vi "1.dé_electronique_Led_Boucle_GJE.vi"() -> ()   [LabVIEW 2018]
panel:
  in  "Numérique":i8=1 min=1 max=6
  out "7":bool
  out "3":bool
  out "2":bool
  out "6":bool
  out "4":bool
  out "1":bool
  out "5":bool
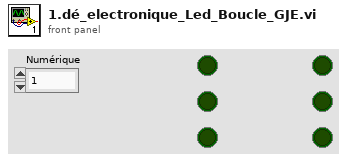
[diagram p1: front panel]
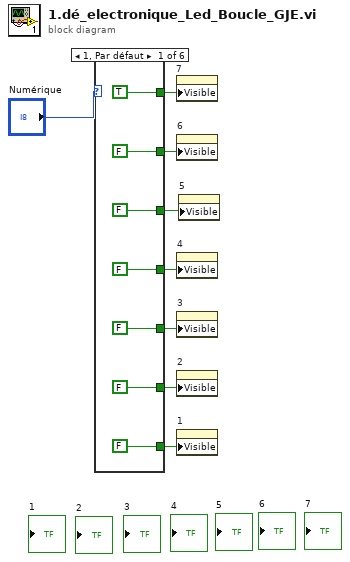
[diagram p0: block diagram]
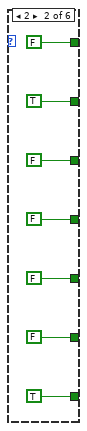
[diagram p2: hidden frame]
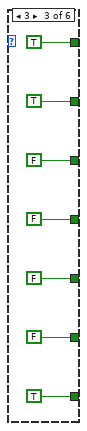
[diagram p3: hidden frame]
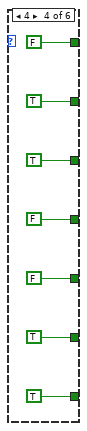
[diagram p4: hidden frame]
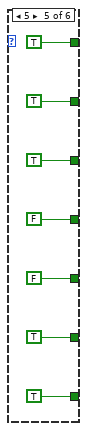
[diagram p5: hidden frame]
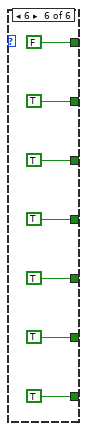
[diagram p6: hidden frame]
diagram:
  n1 = case shown="1, Par défaut" "Numérique" {
    tunnel: [TRUE FALSE TRUE FALSE TRUE FALSE] -> w4
    tunnel: [FALSE TRUE TRUE TRUE TRUE TRUE] -> w3
    tunnel: [FALSE FALSE FALSE TRUE TRUE TRUE] -> w1
    tunnel: [FALSE FALSE FALSE FALSE FALSE TRUE] -> w5
    tunnel: [FALSE FALSE FALSE FALSE FALSE TRUE] -> w6
    tunnel: [FALSE FALSE FALSE TRUE TRUE TRUE] -> w7
    tunnel: [FALSE TRUE TRUE TRUE TRUE TRUE] -> w8
    frame 1, Default {
    }
    frame 2 {
    }
    frame 3 {
    }
    frame 4 {
    }
    frame 5 {
    }
    frame 6 {
    }
  }
  n2 = property on="7" class="Bool (strict)"("Visible"=w4) -> ()  [unwired: 2 in, 2 out]
  n3 = property on="6" class="Bool (strict)"("Visible"=w3) -> ()  [unwired: 2 in, 2 out]
  n4 = property on="4" class="Bool (strict)"("Visible"=w5) -> ()  [unwired: 2 in, 2 out]
  n5 = property on="3" class="Bool (strict)"("Visible"=w6) -> ()  [unwired: 2 in, 2 out]
  n6 = property on="2" class="Bool (strict)"("Visible"=w7) -> ()  [unwired: 2 in, 2 out]
  n7 = property on="1" class="Bool (strict)"("Visible"=w8) -> ()  [unwired: 2 in, 2 out]
  n8 = property on="5" class="Bool (strict)"("Visible"=w1) -> ()  [unwired: 2 in, 2 out]
